vi "GCMSection.vi"() -> ()   [LabVIEW 2014, in "GCMConfigurationManager.lvclass"]
uses:
  GCMConfigurationManager.lvclass
panel:
  in  "GCMSection":string="GCM"
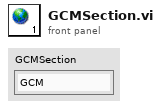
[diagram p1: front panel]
diagram:
